vi "ReadAnalogTask.vi"(6 "error out 2":errorcluster, 9 "Cancel Button":bool) -> (0 "error out 3":errorcluster)   [LabVIEW 2020]
uses:
  <vilib>/DAQmx/read.llb/DAQmx Read (Analog DBL 1Chan 1Samp).vi
  <vilib>/DAQmx/create/channels.llb/DAQmx Create Channel (AI-Voltage-Basic).vi
  <vilib>/DAQmx/configure/timing.llb/DAQmx Timing (Sample Clock).vi
  <vilib>/DAQmx/miscellaneous.llb/DAQmx Fill In Error Info.vi
panel:
  out "Waveform Chart - Dark":dbl(graph)
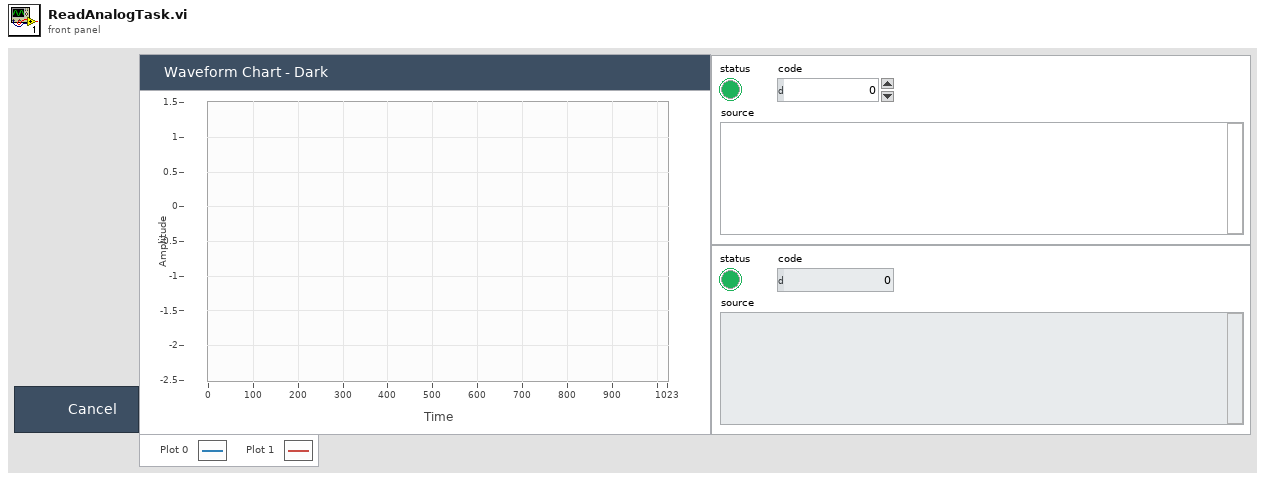
[diagram p1: front panel]
types:
  T1 = enum16{"Create Task", "Sample Rate", "Stop / Clear", "Start Reading"}
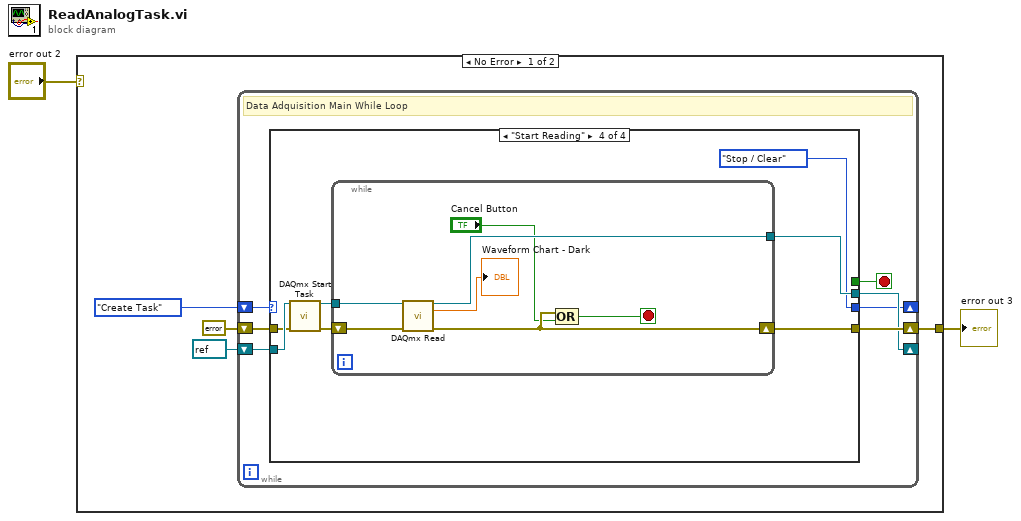
[diagram p0: block diagram]
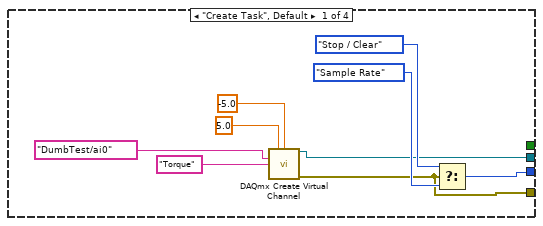
[diagram p2: hidden frame]
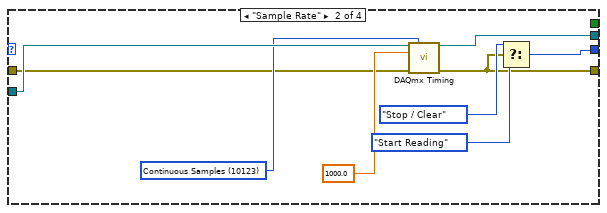
[diagram p3: hidden frame]
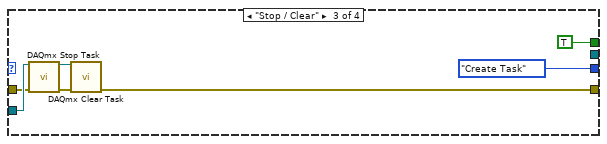
[diagram p4: hidden frame]
diagram:
  n1 = case shown="No Error" "error out 2" {
    tunnel: [w5 _] -> w1
    frame No Error {
      n2 = while {
        shift-right: [w8] -> _
        shift-left: T1."Create Task" -> [w13]
        shift-right: [w9] -> _
        shift-left: refnum<k21> refnum ("task out") -> [w12]
        shift-right: [w10] -> w5
        shift-left: errorcluster {"status"=FALSE, "code"=0, "source"=""} ("error out") -> [w11]
        stop <- w7 stop-if-true
        # "Data Adquisition Main While Loop"
        n3 = case shown="\"Start Reading\"" w13 {
          tunnel: w12 -> [_ w31 w38 w45]
          tunnel: w11 -> [_ w26 w37 w44]
          tunnel: [w16 w25 w34 w41] -> w10
          tunnel: [w17 w24 _ w42] -> w9
          tunnel: [w20 w23 T1."Create Task" T1."Stop / Clear"] -> w8
          tunnel: [_ _ TRUE _] -> w7
          frame "Create Task", Default {
            n4 = call-poly <vilib>:"DAQmx Create Virtual Channel.vi"("maximum value"=5.0, "minimum value"=-5.0, "physical channels"=tag "DumbTest/ai0", "name to assign"="Torque") -> ("task out"=w17:refnum<k21>, "error out"=w16:errorcluster)  [unwired: 10 in]
            n5 = Select(t=T1."Stop / Clear", s=w16, f=T1."Sample Rate") -> (s? t:f=w20:T1)
          }
          frame "Sample Rate" {
            w30 = 10123 items=["Finite Samples"=10178, "Continuous Samples"=10123, "Hardware Timed Single Point"=12522] ("sample mode")
            n6 = call-poly <vilib>:"DAQmx Timing.vi"("task/channels in"=w31, "sample mode"=w30, "rate"=1000.0, "error in"=w26) -> ("task out"=w24:refnum<k21>, "error out"=w25:errorcluster)  [unwired: 10 in]
            n7 = Select(t=T1."Stop / Clear", s=w25, f=T1."Start Reading") -> (s? t:f=w23:T1)
          }
          frame "Stop / Clear" {
            n8 = call <vilib>:"DAQmx Stop Task.vi"("task/channels in"=w38, "error in"=w37) -> ("task out"=w36:refnum<k21>, "error out"=w35:errorcluster)  [unwired: 12 in]
            n9 = call <vilib>:"DAQmx Clear Task.vi"("task in"=w36, "error in"=w35) -> ("error out"=w34:errorcluster)  [unwired: 13 in]
          }
          frame "Start Reading" {
            n10 = call <vilib>:"DAQmx Start Task.vi"("task/channels in"=w45, "error in"=w44) -> ("task out"=w43:refnum<k21>, "error out"=w39:errorcluster)  [unwired: 12 in]
            n11 = while {
              tunnel: w43 -> [w52]
              tunnel: [w50] -> w42
              shift-right: [w49] -> w41
              shift-left: w39 -> [w46]
              stop <- w47 stop-if-true
              n12 = call-poly <vilib>:"DAQmx Read.vi"("task/channels in"=w52, "error in"=w46) -> ("task out"=w50:refnum<k21>, "data"=→"Waveform Chart - Dark":dbl, "error out"=w49:errorcluster)  [unwired: 11 in]
              n13 = Compound Arithmetic op=OR(w49, "Cancel Button") -> (w47:bool)
            }
          }
        }
      }
    }
    frame Error {
    }
  }
  "error out 3" <- w1
